vi "Read All Enqueuers.vi"(8 "error in (no error)":errorcluster, 11 "ExperimentService in":refnum<class "ExperimentService.lvclass">) -> (0 "error out":errorcluster, 2 "Enqueuers":T1, 3 "ExperimentService out":refnum<class "ExperimentService.lvclass">)   [LabVIEW 2014, in "ExperimentService.lvclass"]
uses:
  ExperimentService.lvclass
  <vilib>/ActorFramework/Message Enqueuer/Message Enqueuer.lvclass
  ExperimentService.lvclass/ExperimentService.ctl
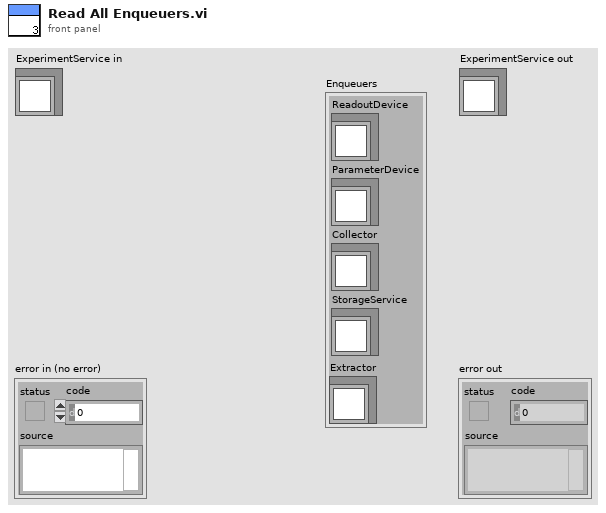
[diagram p1: front panel]
types:
  T1 = cluster{"ReadoutDevice":refnum<class "Message Enqueuer.lvclass">, "ParameterDevice":refnum<class "Message Enqueuer.lvclass">, "Collector":refnum<class "Message Enqueuer.lvclass">, "StorageService":refnum<class "Message Enqueuer.lvclass">, "Extractor":refnum<class "Message Enqueuer.lvclass">}
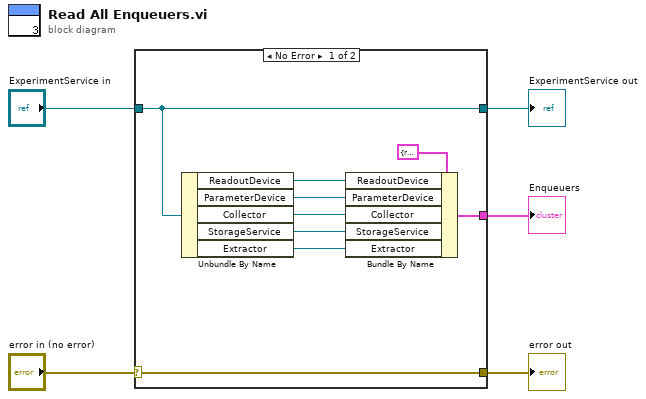
[diagram p0: block diagram]
diagram:
  n1 = case shown="No Error" "error in (no error)" {
    selector: "error in (no error)" -> [w14 w16]
    tunnel: [w14 w16] -> w4
    tunnel: [w13 w15] -> w2
    tunnel: "ExperimentService in" -> [w13 w15]
    tunnel: [w7 _] -> w1
    frame No Error {
      n2 = Unbundle By Name(w13) -> ("ReadoutDevice"=w11:refnum<class "Message Enqueuer.lvclass">, "ParameterDevice"=w10:refnum<class "Message Enqueuer.lvclass">, "Collector"=w9:refnum<class "Message Enqueuer.lvclass">, "StorageService"=w8:refnum<class "Message Enqueuer.lvclass">, "Extractor"=w6:refnum<class "Message Enqueuer.lvclass">)
      n3 = Bundle By Name(cluster=T1 {"ReadoutDevice"=refnum, "ParameterDevice"=refnum, "Collector"=refnum, "StorageService"=refnum, "Extractor"=refnum} ("output cluster"), "ReadoutDevice"=w11, "ParameterDevice"=w10, "Collector"=w9, "StorageService"=w8, "Extractor"=w6) -> (w7:T1)
    }
    frame Error {
    }
  }
  "error out" <- w4
  "ExperimentService out" <- w2
  "Enqueuers" <- w1
